vi "ROI grp-Update group number.vi"(11 "[Groups]":T1[](array[typedef])) -> (3 "[Groups]":T1[](array[typedef]))   [LabVIEW 2013]
uses:
  Typedefs/Group sel cluster.ctl
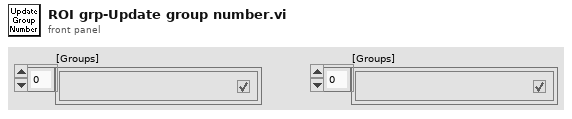
[diagram p1: front panel]
types:
  T1 = typedef "Group sel cluster.ctl" = cluster{"Group number":string, "Group Name":string, "Visibility":bool, "Highlight":bool}
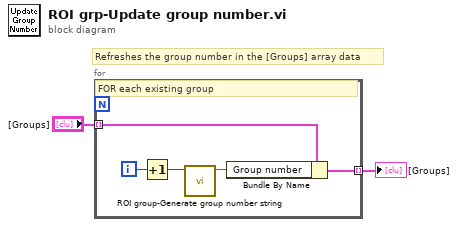
[diagram p0: block diagram]
diagram:
  # "Refreshes the group number in the [Groups] array data"
  n1 = for {
    tunnel: "[Groups]" -> [w5] mode=indexing
    tunnel: [w7] -> w2 mode=indexing
    i -> [w6]
    # "FOR each existing group"
    n2 = Increment(x=w6) -> (x+1=w4:i32)
    n3 = call "ROI group-Generate group number string.vi"("Group number"=w4) -> ("Group number string"=w3:string)  [unwired: 10 in]
    n4 = Bundle By Name(cluster=w5, "Group number"=w3) -> (w7:T1)
  }
  "[Groups]" <- w2
